vi "Render.vi"(8 "error in (no error)":errorcluster, 11 "XRay Beam in":refnum<class "XRay Beam.lvclass">=refnum) -> (0 "error out":errorcluster, 2 "Scene Object":refnum<vi>, 3 "XRay Beam out":refnum<class "XRay Beam.lvclass">)   [LabVIEW 2026, in "XRay Beam.lvclass"]
uses:
  XRay Beam.lvclass
  XRay CArm/XRay CArm.lvclass
  <vilib>/picture/3D Picture Control/Old 3D Toolkit.llb/point3f.ctl
  XRay Beam.lvclass/XRay Beam.ctl
  <vilib>/picture/3D Picture Control/Object/Create Object (name).vi
  <vilib>/picture/3D Picture Control/Object/Add Object (no reference).vi
  3D utilities/3D utilities.lvlib
  <vilib>/picture/3D Picture Control/NI_3D Picture Control.lvlib
  <vilib>/picture/3D Picture Control/NI_Old 3D Toolkit.lvlib
panel:
  in  "Draw Style:Mode":T1(ring)=enum."Wireframe"
  in  "Euler Angles":cluster{"phi":dbl, "theta":dbl, "psi":dbl}
  in  "point3f - SHIFT":T2={"x"=5.5, "y"=1.75, "z"=0.0} {"z" format="%.2f"; "y" format="%.2f"; "x" format="%.2f"}
  in  "DDA SIZE":sgl(slide)=2.0 scale=1.0..4.0
  in  "FDD":sgl(slide)=10.0 scale=1.0..15.0
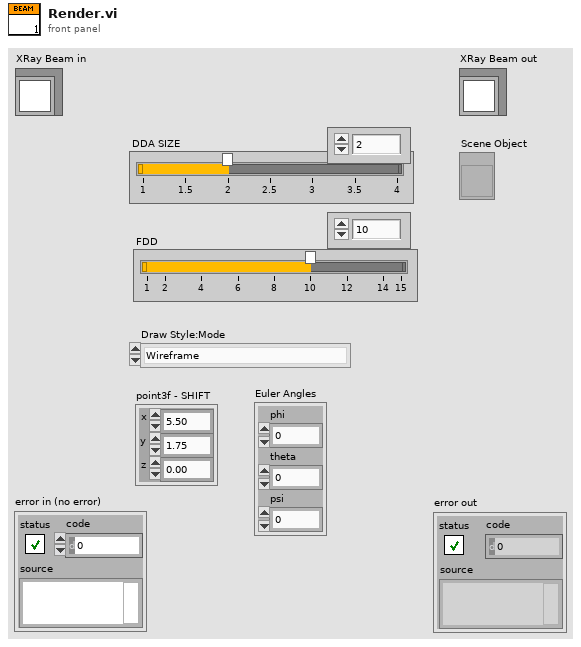
[diagram p1: front panel]
types:
  T1 = enum16{"Inherit Value", "Points", "Wireframe", "Polygons"}
  T2 = typedef "NI_3D Picture Control.lvlib/NI_Old 3D Toolkit.lvlib/point3f.ctl" = cluster{"x":sgl, "y":sgl, "z":sgl}
  T3 = typedef "NI_3D Picture Control.lvlib/NI_Old 3D Toolkit.lvlib/model.ctl" = cluster{"VertexList":T2[], "FaceList":cluster{"v1":i32, "v2":i32, "v3":i32}[], "NormalList":T2[], "Mode":T4}
  T4 = typedef "NI_3D Picture Control.lvlib/NI_Old 3D Toolkit.lvlib/VertexMode.ctl" = enum16{"GL_POINTS", "GL_LINES", "GL_LINE_LOOP", "GL_LINE_STRIP", "GL_TRIANGLES", "GL_TRIANGLE_STRIP", "GL_TRIANGLE_FAN", "GL_QUADS", "GL_QUAD_STRIP", "GL_POLYGON"}
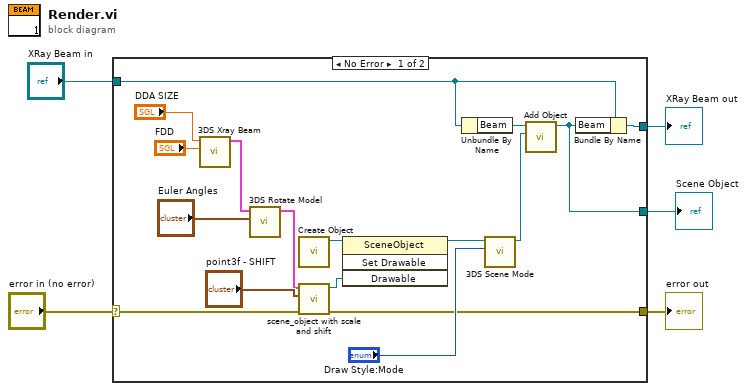
[diagram p0: block diagram]
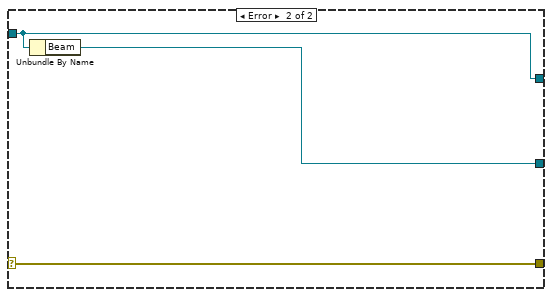
[diagram p2: hidden frame]
diagram:
  n1 = case shown="No Error" "error in (no error)" {
    selector: "error in (no error)" -> [w7 w25]
    tunnel: [w6 w25] -> w4
    tunnel: [w9 w24] -> w2
    tunnel: "XRay Beam in" -> [w10 w24]
    tunnel: [w8 w23] -> w1
    frame No Error {
      n2 = call "3DS Xray Beam.vi"("FDD"="FDD", "DETECTOR SIZE"="DDA SIZE") -> ("XRAY BEAM"=w19:T3)  [unwired: 9 in]
      n3 = call "3DS Rotate Model.vi"("Euler Angles"="Euler Angles", "model in"=w19) -> ("model out"=w18:T3)  [unwired: 9 in]
      n4 = call-poly <vilib>:"Create Object.vi"() -> ("Scene:New Object"=w16:refnum<vi>)  [unwired: 10 in, 1 out]
      n5 = call "scene_object with scale and shift.vi"("error in (no error)"=w7, "point3f - SHIFT"="point3f - SHIFT", "Object In"=w18) -> ("error out"=w6:errorcluster, "SceneMesh out"=w15:refnum<vi>)  [unwired: 4 in, 3 out]
      n6 = invoke class="SceneObject" method="Set Drawable"(reference=w16, "Drawable"=w15) -> (reference out=w14:refnum<vi>)  [unwired: 2 in, 3 out]
      n7 = Unbundle By Name(w10) -> ("Beam"=w12:refnum<vi>)
      n8 = call "3DS Scene Mode.vi"("Draw Style:Mode"="Draw Style:Mode", "SceneObject in"=w14) -> ("SceneObject out"=w11:refnum<vi>)  [unwired: 8 in, 1 out]
      n9 = call-poly <vilib>:"Add Object.vi"("New Object In"=w11, "Scene Object In"=w12) -> ("Scene Object Out"=w8:refnum<vi>)  [unwired: 8 in, 1 out]
      n10 = Bundle By Name(cluster=w10, "Beam"=w8) -> (w9:refnum<class "XRay Beam.lvclass">)
    }
    frame Error {
      n11 = Unbundle By Name(w24) -> ("Beam"=w23:refnum<vi>)
    }
  }
  "error out" <- w4
  "XRay Beam out" <- w2
  "Scene Object" <- w1
